vi "JUnit Aggregate.vi"() -> ()   [LabVIEW 2013]
doc: "This example illustrates how multiple test suites can be combined in one aggregate JUnit XML report."
uses:
  JUnit XML/Test Suites/Test Suites.lvclass
  <vilib>/xml/Close Reference(Node).vi
  <vilib>/xml/NI_XML.lvlib
  <resource>/objmgr/DOMUserDefRef.rc
  JUnit XML/Test Case/Test Case.lvclass
  JUnit XML/Test Suite/Test Suite.lvclass
panel:
  out "XML":string
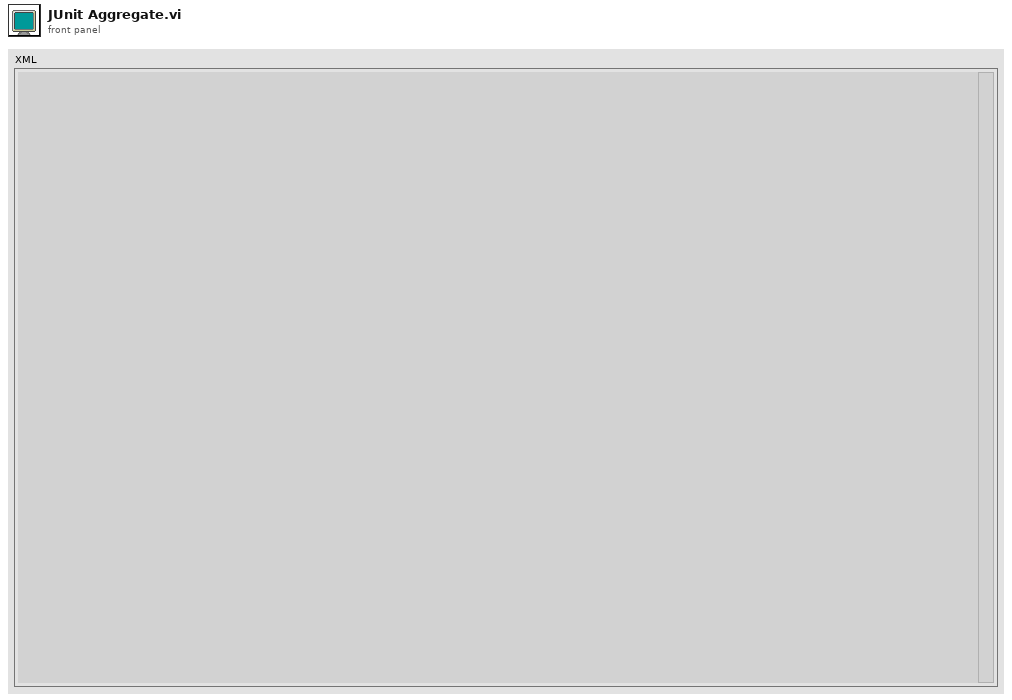
[diagram p1: front panel]
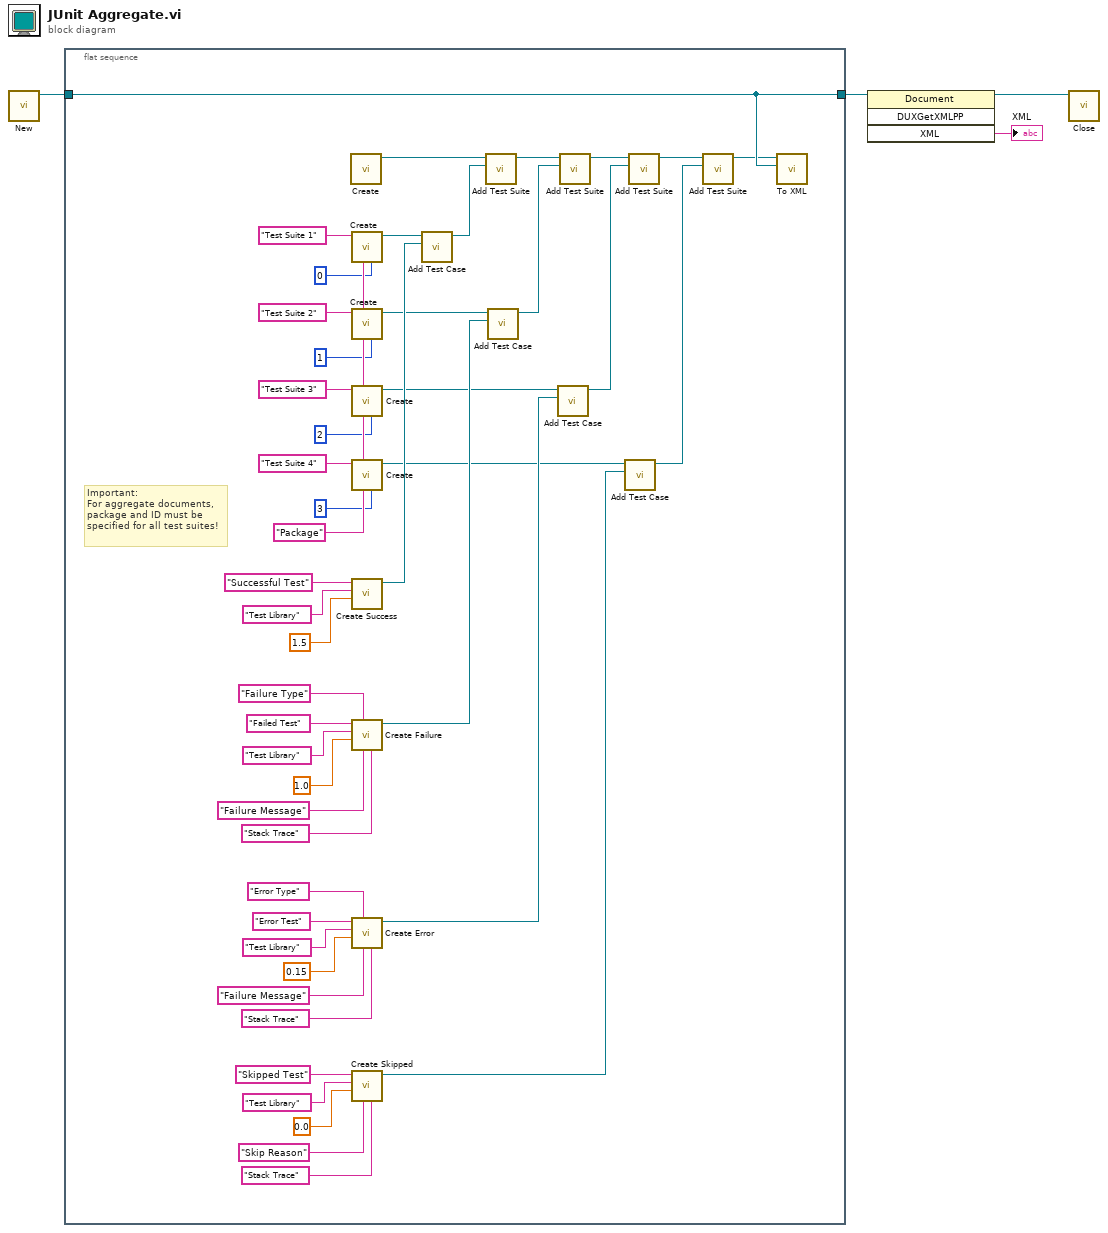
[diagram p0: block diagram]
diagram:
  n1 = call <vilib>:"New.vi"() -> ("DOM document out"=w4:refnum<k20>)  [unwired: 8 in, 1 out]
  n2 = flat-sequence {
    tunnel: w4 -> [w45]
    tunnel: [w45] -> w2
    frame #0 {
      w9 = "Package" ("Package (\"\" = undefined)")
      # "Important:\nFor aggregate documents,\npackage and ID must be\nspecified for all test suites!"
      n3 = call "Create.vi"() -> ("Test Suites"=w24:refnum<class "Test Suites.lvclass">)  [unwired: 10 in, 1 out]
      n4 = call "Create.vi"("Id (-1 = undefined)"=0, "Package (\"\" = undefined)"=w9, "Name"="Test Suite 1") -> ("Test Suite"=w47:refnum<class "Test Suite.lvclass">)  [unwired: 7 in, 1 out]
      n5 = call "Create.vi"("Id (-1 = undefined)"=1, "Package (\"\" = undefined)"=w9, "Name"="Test Suite 2") -> ("Test Suite"=w19:refnum<class "Test Suite.lvclass">)  [unwired: 7 in, 1 out]
      n6 = call "Create.vi"("Id (-1 = undefined)"=2, "Package (\"\" = undefined)"=w9, "Name"="Test Suite 3") -> ("Test Suite"=w18:refnum<class "Test Suite.lvclass">)  [unwired: 7 in, 1 out]
      n7 = call "Create.vi"("Id (-1 = undefined)"=3, "Package (\"\" = undefined)"=w9, "Name"="Test Suite 4") -> ("Test Suite"=w17:refnum<class "Test Suite.lvclass">)  [unwired: 7 in, 1 out]
      n8 = call "Create Success.vi"("Time"=1.5, "Classname"="Test Library", "Name"="Successful Test") -> ("Test Case"=w46:refnum<class "Test Case.lvclass">)  [unwired: 7 in, 1 out]
      n9 = call "Create Failure.vi"("Stack Trace"="Stack Trace", "Message"="Failure Message", "Type"="Failure Type", "Time"=1.0, "Classname"="Test Library", "Name"="Failed Test") -> ("Test Case"=w38:refnum<class "Test Case.lvclass">)  [unwired: 4 in, 1 out]
      n10 = call "Create Error.vi"("Stack Trace"="Stack Trace", "Message"="Failure Message", "Type"="Error Type", "Time"=0.15, "Classname"="Test Library", "Name"="Error Test") -> ("Test Case"=w31:refnum<class "Test Case.lvclass">)  [unwired: 4 in, 1 out]
      n11 = call "Create Skipped.vi"("Stack Trace"="Stack Trace", "Message"="Skip Reason", "Time"=0.0, "Classname"="Test Library", "Name"="Skipped Test") -> ("Test Case"=w25:refnum<class "Test Case.lvclass">)  [unwired: 5 in, 1 out]
      n12 = call "Add Test Case.vi"("Test Case"=w46, "Test Suite in"=w47) -> ("Test Suite out"=w23:refnum<class "Test Suite.lvclass">)  [unwired: 8 in, 1 out]
      n13 = call "Add Test Suite.vi"("Test Suite"=w23, "Test Suites in"=w24) -> ("Test Suites out"=w16:refnum<class "Test Suites.lvclass">)  [unwired: 8 in, 1 out]
      n14 = call "Add Test Case.vi"("Test Case"=w38, "Test Suite in"=w19) -> ("Test Suite out"=w15:refnum<class "Test Suite.lvclass">)  [unwired: 8 in, 1 out]
      n15 = call "Add Test Case.vi"("Test Case"=w31, "Test Suite in"=w18) -> ("Test Suite out"=w14:refnum<class "Test Suite.lvclass">)  [unwired: 8 in, 1 out]
      n16 = call "Add Test Suite.vi"("Test Suite"=w15, "Test Suites in"=w16) -> ("Test Suites out"=w13:refnum<class "Test Suites.lvclass">)  [unwired: 8 in, 1 out]
      n17 = call "Add Test Case.vi"("Test Case"=w25, "Test Suite in"=w17) -> ("Test Suite out"=w12:refnum<class "Test Suite.lvclass">)  [unwired: 8 in, 1 out]
      n18 = call "Add Test Suite.vi"("Test Suite"=w14, "Test Suites in"=w13) -> ("Test Suites out"=w11:refnum<class "Test Suites.lvclass">)  [unwired: 8 in, 1 out]
      n19 = call "Add Test Suite.vi"("Test Suite"=w12, "Test Suites in"=w11) -> ("Test Suites out"=w10:refnum<class "Test Suites.lvclass">)  [unwired: 8 in, 1 out]
      n20 = call-dynamic "To XML.vi"("Parent"=w45, "Test Suites in"=w10) -> ()  [unwired: 9 in, 1 out]
    }
  }
  n21 = invoke class="Document" method="DUXGetXMLPP"(reference=w2) -> (reference out=w3:refnum<k20>, "XML"=→"XML":string)  [unwired: 3 in, 2 out]
  n22 = call-poly <vilib>:"Close.vi"("node"=w3) -> ()  [unwired: 8 in, 1 out]
